vi "carwash_test2.vi"() -> ()   [LabVIEW 2017]
panel:
  out "?":bool
  in  "?":bool
  out "?":bool
  out "?":bool
  in  "Wash Selec.":enum16{"Initialize", "Deluxe", "Economy"}(ring)
  out "Vehicle Out of Position":bool=TRUE
  out "Air Dry":bool
  out "Clear Water Rinse":bool
  out "Main High Press. Wash":bool
  out "Soap Application":bool
  out "Under body Wash":bool
  in  "?":bool
  in  "?":bool
  in  "stop":bool
  # "Car Wash Indicators"
  # "Underbody wash\nposition \nSwitch"
  # "Main Wash \nPosition \nSwitch"
  # "Air Dry\nPosition\nSwitch"
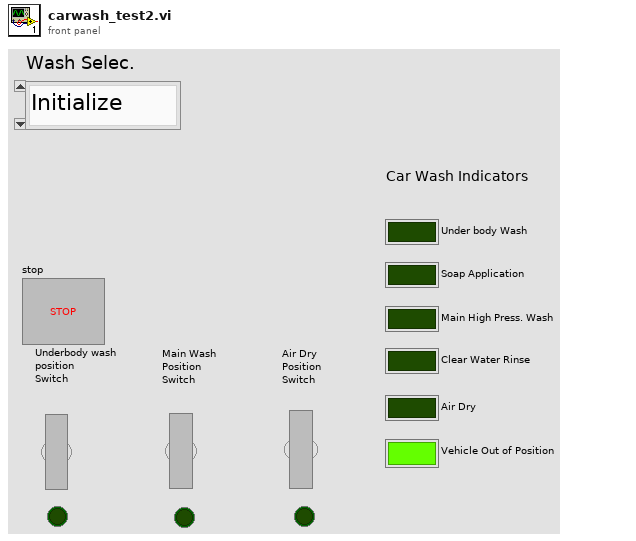
[diagram p1: front panel]
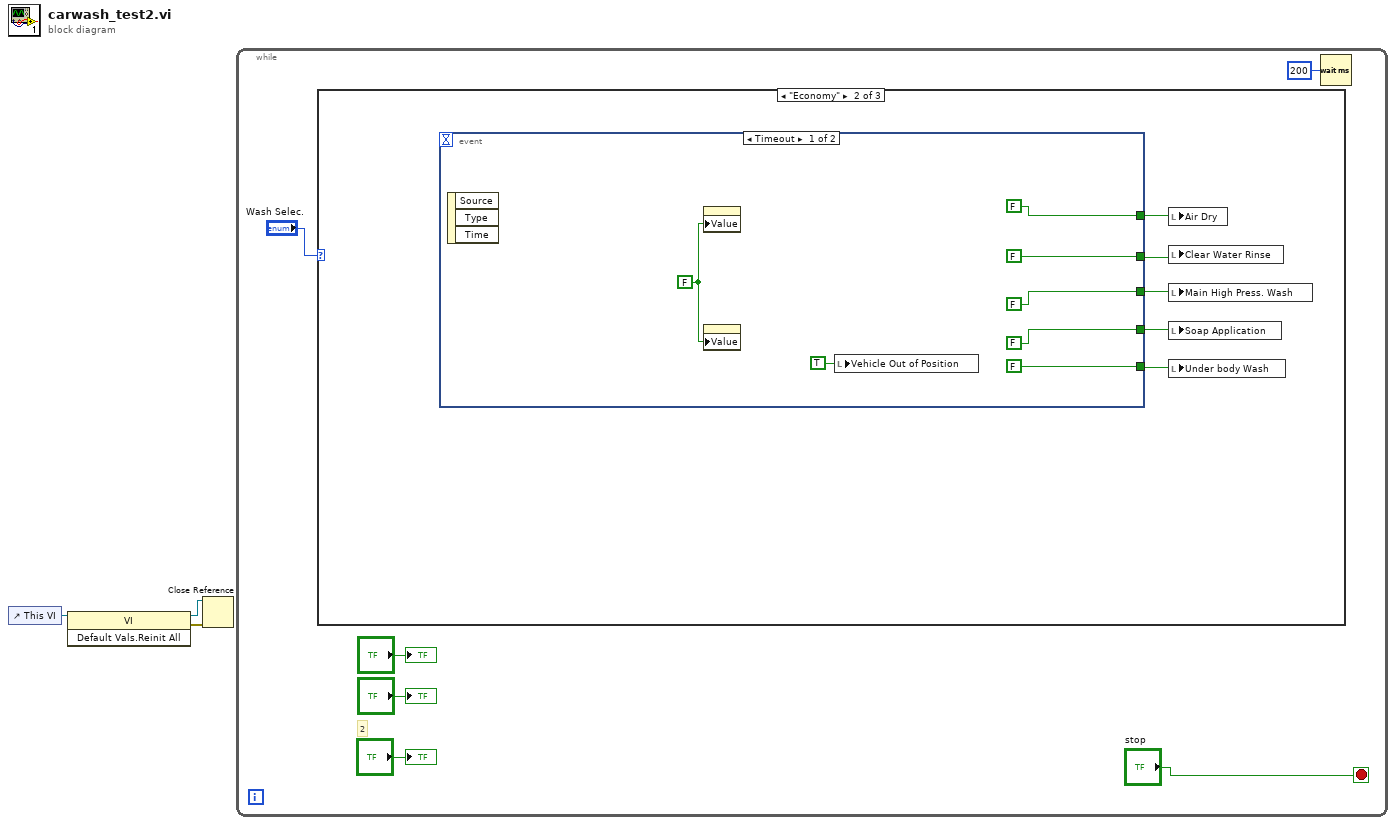
[diagram p0: block diagram]
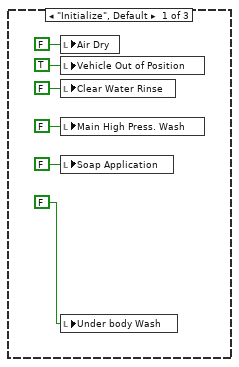
[diagram p2: hidden frame]
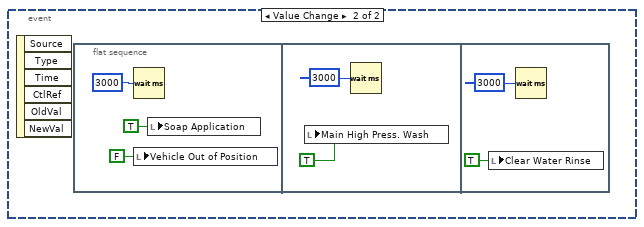
[diagram p3: hidden frame]
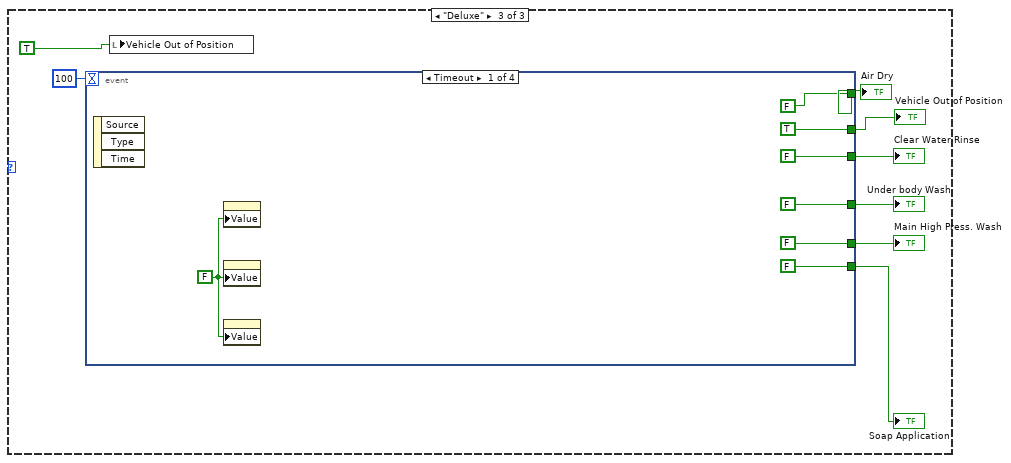
[diagram p4: hidden frame]
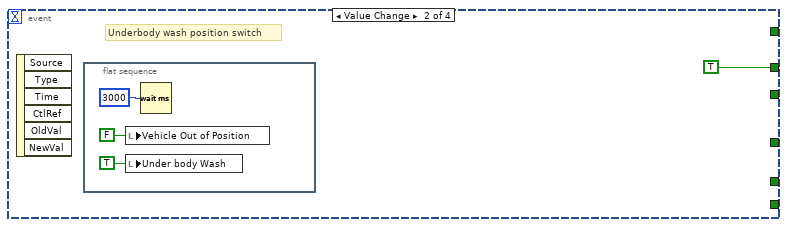
[diagram p5: hidden frame]
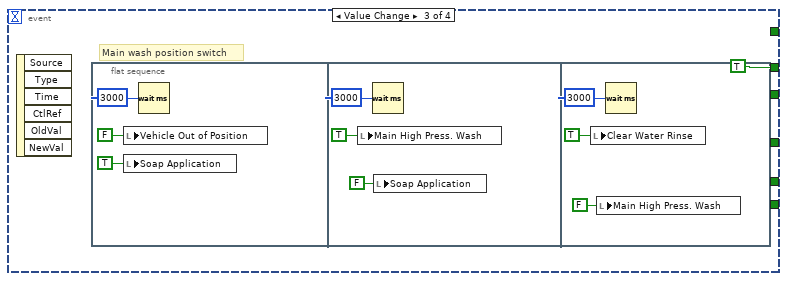
[diagram p6: hidden frame]
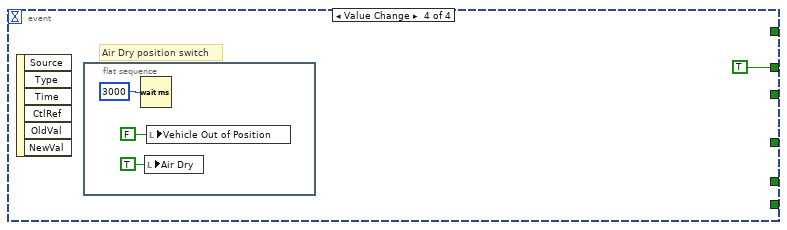
[diagram p7: hidden frame]
diagram:
  n1 = control-ref of="This VI"() -> (w3:refnum<vi>)
  n2 = invoke class="VI" method="Default Vals.Reinit All"(reference=w3) -> (reference out=w2:refnum<vi>, error out=w1:errorcluster)  [unwired: 2 in, 1 out]
  n3 = Close Reference(reference=w2, error in (no error)=w1) -> ()  [unwired: 1 out]
  n4 = while {
    stop <- "stop" stop-if-true
    # "1"
    # "2"
    n5 = case shown="\"Economy\"" "Wash Selec." {
      frame "Initialize", Default {
        n6 = local write "Air Dry"(FALSE) -> ()
        n7 = local write "Vehicle Out of Position"(TRUE) -> ()
        n8 = local write "Clear Water Rinse"(FALSE) -> ()
        n9 = local write "Main High Press. Wash"(FALSE) -> ()
        n10 = local write "Soap Application"(FALSE) -> ()
        n11 = local write "Under body Wash"(FALSE) -> ()
      }
      frame "Economy" {
        n12 = event shown="[0] Timeout" {
          selector: _ -> [_ _]
          dyn-events: _ -> [_ _]
          timeout: _ -> [_ _]
          tunnel: [FALSE _] -> w16
          tunnel: [FALSE _] -> w17
          tunnel: [FALSE _] -> w18
          tunnel: [FALSE _] -> w19
          tunnel: [FALSE _] -> w20
          event Timeout {
            w21 = FALSE
            n13 = event-data() -> ()  [unwired: 1 in, 3 out]
            n14 = property class="Bool (strict)"("Value"=w21) -> ()  [unwired: 2 in, 2 out]
            n15 = property class="Bool (strict)"("Value"=w21) -> ()  [unwired: 2 in, 2 out]
            n16 = local write "Vehicle Out of Position"(TRUE ("Vehicle Out of Position")) -> ()
          }
          event Value Change {
            n17 = event-data() -> ()  [unwired: 1 in, 6 out]
            n18 = flat-sequence {
              frame #0 {
                n19 = Wait (ms)(milliseconds to wait=u32 3000) -> ()  [unwired: 1 out]
                n20 = local write "Vehicle Out of Position"(FALSE ("Vehicle Out of Position")) -> ()
                n21 = local write "Soap Application"(TRUE ("Soap Application")) -> ()
              }
              frame #1 {
                n22 = local write "Main High Press. Wash"(TRUE ("Main High Press. Wash")) -> ()
                n23 = Wait (ms)(milliseconds to wait=u32 3000) -> ()  [unwired: 1 out]
              }
              frame #2 {
                n24 = local write "Clear Water Rinse"(TRUE ("Clear Water Rinse")) -> ()
                n25 = Wait (ms)(milliseconds to wait=u32 3000) -> ()  [unwired: 1 out]
              }
            }
          }
        }
        n26 = local write "Air Dry"(w16) -> ()
        n27 = local write "Clear Water Rinse"(w17) -> ()
        n28 = local write "Main High Press. Wash"(w18) -> ()
        n29 = local write "Soap Application"(w19) -> ()
        n30 = local write "Under body Wash"(w20) -> ()
      }
      frame "Deluxe" {
        n31 = event shown="[0] Timeout" {
          selector: _ -> [_ _ _ _]
          dyn-events: _ -> [_ _ _ _]
          timeout: 100 -> [_ _ _ _]
          tunnel: [FALSE _ _ _] -> w42
          tunnel: [FALSE _ _ _] -> w41
          tunnel: [FALSE _ _ _] -> w40
          tunnel: [FALSE _ _ _] -> w39
          tunnel: [FALSE _ _ _] -> w38
          tunnel: [TRUE TRUE TRUE TRUE] -> w37
          event Timeout {
            w43 = FALSE
            n32 = event-data() -> ()  [unwired: 1 in, 3 out]
            n33 = property class="Bool (strict)"("Value"=w43) -> ()  [unwired: 2 in, 2 out]
            n34 = property class="Bool (strict)"("Value"=w43) -> ()  [unwired: 2 in, 2 out]
            n35 = property class="Bool (strict)"("Value"=w43) -> ()  [unwired: 2 in, 2 out]
          }
          event Value Change {
            # "Underbody wash position switch"
            n36 = event-data() -> ()  [unwired: 1 in, 6 out]
            n37 = flat-sequence {
              frame #0 {
                n38 = local write "Vehicle Out of Position"(FALSE ("Vehicle Out of Position")) -> ()
                n39 = local write "Under body Wash"(TRUE ("Under body Wash")) -> ()
                n40 = Wait (ms)(milliseconds to wait=u32 3000) -> ()  [unwired: 1 out]
              }
            }
          }
          event Value Change {
            # "Main wash position switch"
            n41 = event-data() -> ()  [unwired: 1 in, 6 out]
            n42 = flat-sequence {
              frame #0 {
                n43 = local write "Vehicle Out of Position"(FALSE ("Vehicle Out of Position")) -> ()
                n44 = local write "Soap Application"(TRUE ("Boolean 2")) -> ()
                n45 = Wait (ms)(milliseconds to wait=u32 3000) -> ()  [unwired: 1 out]
              }
              frame #1 {
                n46 = local write "Main High Press. Wash"(TRUE ("Boolean 4")) -> ()
                n47 = Wait (ms)(milliseconds to wait=u32 3000) -> ()  [unwired: 1 out]
                n48 = local write "Soap Application"(FALSE ("Soap Application")) -> ()
              }
              frame #2 {
                n49 = local write "Clear Water Rinse"(TRUE ("Boolean 4")) -> ()
                n50 = local write "Main High Press. Wash"(FALSE ("Main High Press. Wash")) -> ()
                n51 = Wait (ms)(milliseconds to wait=u32 3000) -> ()  [unwired: 1 out]
              }
            }
          }
          event Value Change {
            # "Air Dry position switch"
            n52 = event-data() -> ()  [unwired: 1 in, 6 out]
            n53 = flat-sequence {
              frame #0 {
                n54 = Wait (ms)(milliseconds to wait=u32 3000) -> ()  [unwired: 1 out]
                n55 = local write "Air Dry"(TRUE ("Air Dry")) -> ()
                n56 = local write "Vehicle Out of Position"(FALSE ("Vehicle Out of Position")) -> ()
              }
            }
          }
        }
        "Under body Wash" <- w42
        "Soap Application" <- w41
        "Main High Press. Wash" <- w40
        "Clear Water Rinse" <- w39
        "Air Dry" <- w38
        "Vehicle Out of Position" <- w37
        n57 = local write "Vehicle Out of Position"(TRUE ("Vehicle Out of Position")) -> ()
      }
    }
    n58 = Wait (ms)(milliseconds to wait=u32 200) -> ()  [unwired: 1 out]
    "?" <- "?"
    "?" <- "?"
    "?" <- "?"
  }
